vi "ConfigureTiming.vi"(0 "object in":refnum<class "AD2_MSO_SDK.lvclass">, 5 "error in (no error)":errorcluster) -> (14 "object out":refnum<class "AD2_MSO_SDK.lvclass">, 19 "error out":errorcluster)   [LabVIEW 2024, in "AD2_MSO_SDK.lvclass"]
uses:
  AD2_MSO_SDK.lvclass
  AD2_MSO_SDK.lvclass/AD2_MSO_SDK.ctl
  Olasdwf/Olasdwf.lvlib
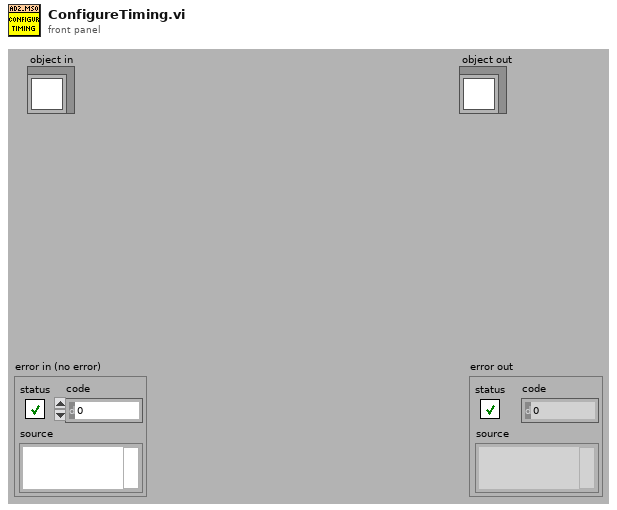
[diagram p1: front panel]
types:
  T1 = enum16{"Single Sample", "Scanshift", "Multiple Samples", "Scan Screen"}
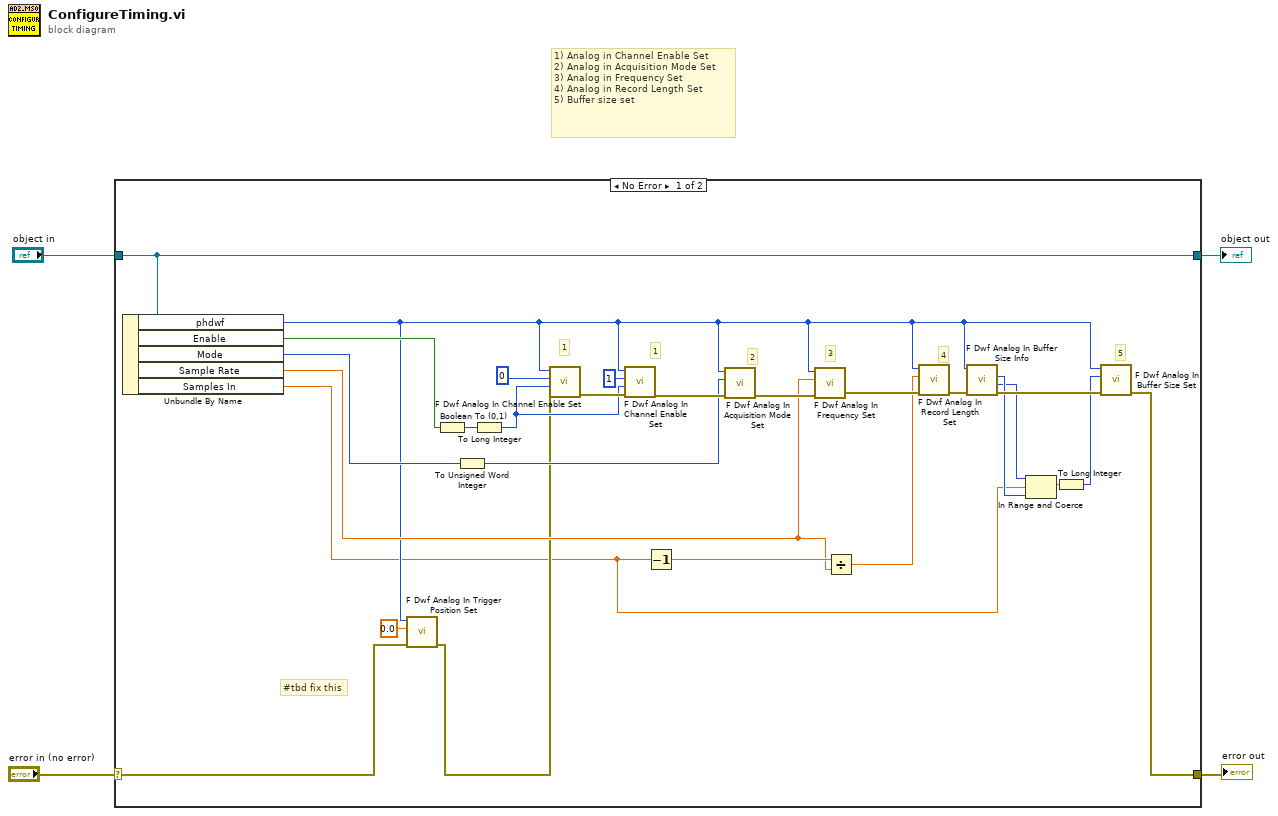
[diagram p0: block diagram]
diagram:
  # "1) Analog in Channel Enable Set\n2) Analog in Acquisition Mode Set\n3) Analog in Frequency Set\n4) Analog in Record Length Set\n5) Buffer size set"
  n1 = case shown="No Error" "error in (no error)" {
    selector: "error in (no error)" -> [w16 w33]
    tunnel: [w11 w33] -> w3
    tunnel: [w31 w32] -> w1
    tunnel: "object in" -> [w31 w32]
    frame No Error {
      # "5"
      # "#tbd fix this"
      # "4"
      # "3"
      # "2"
      # "1"
      # "1"
      n2 = Unbundle By Name(w31) -> ("phdwf"=w8:i32, "Enable"=w20:bool, "Mode"=w19:T1, "Sample Rate"=w17:dbl, "Samples In"=w7:dbl)
      n3 = call "F Dwf Analog In Trigger Position Set.vi"("error in (no error)"=w16, "secPosition"=0.0, "hdwf"=w8) -> ("error out"=w15:errorcluster)  [unwired: 7 in, 1 out]
      n4 = Boolean To (0,1)(Boolean=w20) -> (0, 1=w28:i16)
      n5 = To Unsigned Word Integer(number=w19) -> (unsigned 16bit integer=w18:u16)
      n6 = To Long Integer(number=w28) -> (32bit integer=w26:i32)
      n7 = call "F Dwf Analog In Channel Enable Set.vi"("error in (no error)"=w15, "fEnable"=w26, "idxChannel"=0, "hdwf"=w8) -> ("error out"=w27:errorcluster)  [unwired: 6 in, 1 out]
      n8 = call "F Dwf Analog In Channel Enable Set.vi"("error in (no error)"=w27, "fEnable"=w26, "idxChannel"=1, "hdwf"=w8) -> ("error out"=w25:errorcluster)  [unwired: 6 in, 1 out]
      n9 = Decrement(x=w7) -> (x-1=w22:dbl)
      n10 = call "F Dwf Analog In Acquisition Mode Set.vi"("error in (no error)"=w25, "acqmode"=w18, "hdwf"=w8) -> ("error out"=w24:errorcluster)  [unwired: 7 in, 1 out]
      n11 = call "F Dwf Analog In Frequency Set.vi"("error in (no error)"=w24, "hzFrequency"=w17, "hdwf"=w8) -> ("error out"=w23:errorcluster)  [unwired: 7 in, 1 out]
      n12 = Divide(x=w22, y=w17) -> (x/y=w21:dbl)
      n13 = call "F Dwf Analog In Record Length Set.vi"("error in (no error)"=w23, "sLength"=w21, "hdwf"=w8) -> ("error out"=w13:errorcluster)  [unwired: 7 in, 1 out]
      n14 = call "F Dwf Analog In Buffer Size Info.vi"("error in (no error)"=w13, "hdwf"=w8) -> ("error out"=w12:errorcluster, "pnSizeMax out"=w9:i32, "pnSizeMin out"=w10:i32)  [unwired: 6 in, 1 out]
      n15 = In Range and Coerce(upper limit=w9, x=w7, lower limit=w10) -> (coerced(x)=w6:dbl)  [unwired: 1 out]
      n16 = To Long Integer(number=w6) -> (32bit integer=w5:i32)
      n17 = call "F Dwf Analog In Buffer Size Set.vi"("error in (no error)"=w12, "nSize"=w5, "hdwf"=w8) -> ("error out"=w11:errorcluster)  [unwired: 7 in, 1 out]
    }
    frame Error {
    }
  }
  "error out" <- w3
  "object out" <- w1
